vi "open_visa_session.vi"(8 "error in (no error)":errorcluster, 10 "Cluster":T1={"Baudrate (9600)"=9600, "Data Bits (8)"=8, "Parity (None)"=0, "Stop Bits (1)"=10, "Flow Control (None)"=0, "End Mode for Reads (TermChar)"=0} {"End Mode for Reads (TermChar)" items=["None", "Last Bit", "TermChar"]; "Flow Control (None)" items=["None", "XON/XOFF", "RTS/CTS", "XON/XOFF & RTS/CTS", "DTR/DSR", "XON/XOFF & DTR/DSR"]; "Stop Bits (1)" items=["1.0"=10, "1.5"=15, "2.0"=20]; "Parity (None)" items=["None", "Odd", "Even", "Mark", "Space"]; "Baudrate (9600)" items=["9600"=9600, "19200"=19200, "115200"=115200]}, 11 "ComPort":refnum<visa-resource-name>="COM1") -> (0 "error out":errorcluster, 3 "VISA resource name out":refnum<visa-resource-name>)   [LabVIEW 2018]
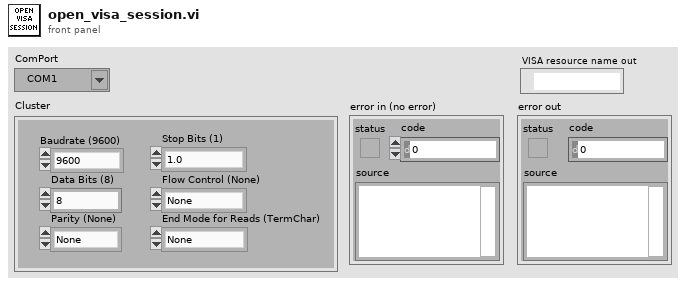
[diagram p1: front panel]
types:
  T1 = cluster{"Baudrate (9600)":u32, "Data Bits (8)":u16, "Parity (None)":u16, "Stop Bits (1)":u16, "Flow Control (None)":u16, "End Mode for Reads (TermChar)":u16}
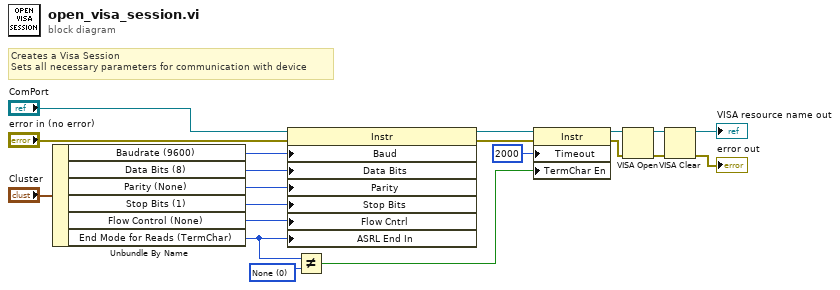
[diagram p0: block diagram]
diagram:
  w3 = u16 0 items=["None", "Last Bit", "TermChar"] ("Serial Settings:End Mode for Reads")
  # "Creates a Visa Session\nSets all necessary parameters for communication with device"
  n1 = Unbundle By Name("Cluster") -> ("Baudrate (9600)"=w8:u32, "Data Bits (8)"=w7:u16, "Parity (None)"=w6:u16, "Stop Bits (1)"=w5:u16, "Flow Control (None)"=w1:u16, "End Mode for Reads (TermChar)"=w4:u16)
  n2 = property class="Instr"(reference="ComPort", error in="error in (no error)", "Baud"=w8, "Data Bits"=w7, "Parity"=w6, "Stop Bits"=w5, "Flow Cntrl"=w1, "ASRL End In"=w4) -> (reference out=w16:refnum<visa-resource-name>, error out=w18:errorcluster)
  n3 = Not Equal?(x=w4, y=w3) -> (x != y?=w2:bool)
  n4 = property class="Instr"(reference=w16, error in=w18, "Timeout"=u32 2000 ("General Settings:Timeout Value"), "TermChar En"=w2) -> (reference out=w15:refnum<visa-resource-name>, error out=w14:errorcluster)
  n5 = VISA Open(error in (no error)=w14, VISA resource name=w15) -> (VISA resource name=w13:refnum<visa-resource-name>, error out=w12:errorcluster)  [unwired: 3 in]
  n6 = VISA Clear(VISA resource name=w13, error in (no error)=w12) -> (VISA resource name out=→"VISA resource name out":refnum<visa-resource-name>, error out=→"error out":errorcluster)
